vi "Align.vi"(6 "Variant in":variant, 7 "Shift Pressed?":bool, 8 "error in (no error)":errorcluster, 10 "QD Combo Box Ref":refnum<vi>, 11 "QD Launch VI Ref":refnum<vi>) -> (0 "error out":errorcluster, 4 "Variant out":variant)   [LabVIEW 2013]
doc: "Default Shortcut - [A]"
panel:
  in  "Undo Name":string="Quick Drop Align"
  # "Do not change the connector pane of this VI.\n\nSee the block diagram for directions on how to use this template."
  # "Specify the name of the Undo transaction"
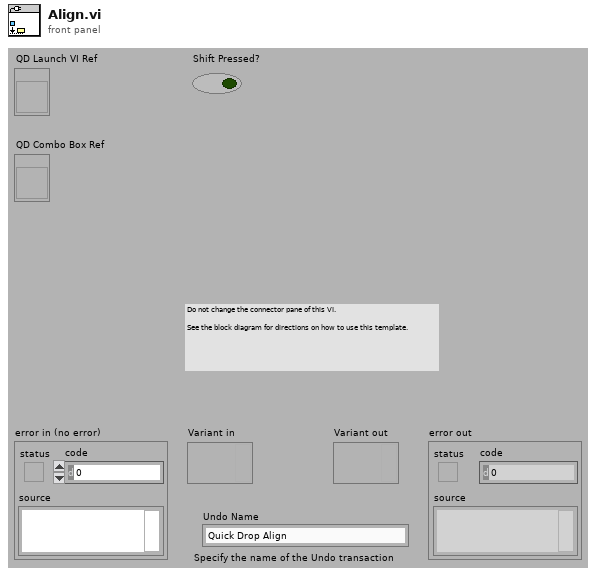
[diagram p1: front panel]
types:
  T1 = enum32{"Top Edges", "Vertical Centers", "Bottom Edges", "Left Edges", "Horizontal Centers", "Right Edges"}
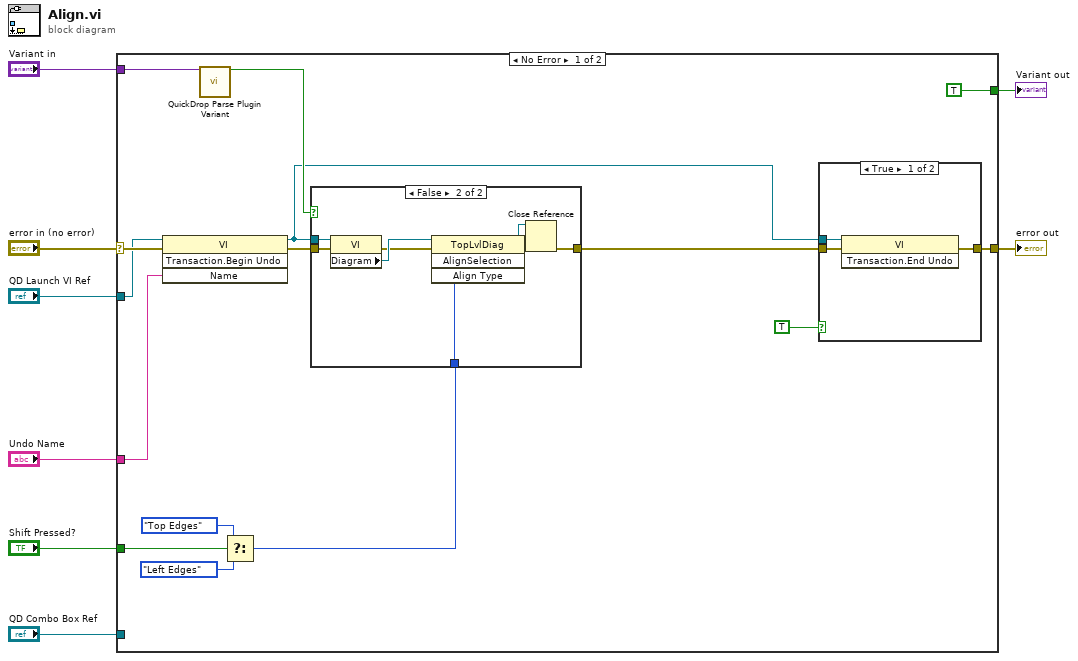
[diagram p0: block diagram]
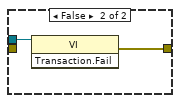
[diagram p2: hidden frame]
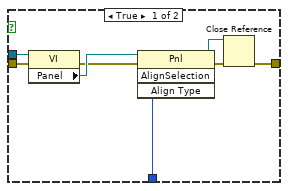
[diagram p3: hidden frame]
diagram:
  n1 = case shown="No Error" "error in (no error)" {
    selector: "error in (no error)" -> [w22 w45]
    tunnel: [w16 w45] -> w7
    tunnel: "QD Launch VI Ref" -> [w21 _]
    tunnel: "Shift Pressed?" -> [w12 _]
    tunnel: "QD Combo Box Ref" -> [_ _]
    tunnel: "Variant in" -> [w23 _]
    tunnel: "Undo Name" -> [w20 _]
    tunnel: [TRUE _] -> w1
    frame No Error {
      n2 = invoke class="VI" method="Transaction.Begin Undo"(reference=w21, error in=w22, "Name"=w20) -> (reference out=w15:refnum<vi>, error out=w17:errorcluster)  [unwired: 1 in, 2 out]
      n3 = call <vilib>:"QuickDrop Parse Plugin Variant.vi"("QDKS Variant in"=w23) -> ("QD Launch VI Panel?"=w18:bool)  [unwired: 12 in, 2 out]
      n4 = Select(t=T1."Top Edges" ("Align Type"), s=w12, f=T1."Left Edges" ("Align Type")) -> (s? t:f=w10:T1)
      n5 = case shown="False" w18 {
        tunnel: w17 -> [w36 w44]
        tunnel: w15 -> [w35 w43]
        tunnel: w10 -> [w30 w38]
        tunnel: [w29 w37] -> w9
        frame True {
          n6 = property class="VI"(reference=w35, error in=w36) -> (error out=w33:errorcluster, "Panel"=w34:refnum<vi>)  [unwired: 1 out]
          n7 = invoke class="Pnl" method="AlignSelection"(reference=w34, error in=w33, "Align Type"=w30) -> (reference out=w31:refnum<vi>, error out=w32:errorcluster)  [unwired: 1 in, 2 out]
          n8 = Close Reference(reference=w31, error in (no error)=w32) -> (error out=w29:errorcluster)
        }
        frame False {
          n9 = property class="VI"(reference=w43, error in=w44) -> (error out=w41:errorcluster, "Diagram"=w42:refnum<vi>)  [unwired: 1 out]
          n10 = invoke class="TopLvlDiag" method="AlignSelection"(reference=w42, error in=w41, "Align Type"=w38) -> (reference out=w39:refnum<vi>, error out=w40:errorcluster)  [unwired: 1 in, 2 out]
          n11 = Close Reference(reference=w39, error in (no error)=w40) -> (error out=w37:errorcluster)
        }
      }
      n12 = case shown="True" TRUE {
        tunnel: w15 -> [w25 w27]
        tunnel: [w26 w28] -> w16
        tunnel: w9 -> [w24 _]
        frame True {
          n13 = invoke class="VI" method="Transaction.End Undo"(reference=w25, error in=w24) -> (error out=w26:errorcluster)  [unwired: 1 in, 2 out]
        }
        frame False {
          n14 = invoke class="VI" method="Transaction.Fail"(reference=w27) -> (error out=w28:errorcluster)  [unwired: 2 in, 2 out]
        }
      }
    }
    frame Error {
    }
  }
  "error out" <- w7
  "Variant out" <- w1
